vi "1-1 Constellations.vi"() -> ()   [LabVIEW 2019, in "AoC2022.lvlib"]
uses:
  AoC2022.lvlib
panel:
  out "Array":i32[][](array[numeric])
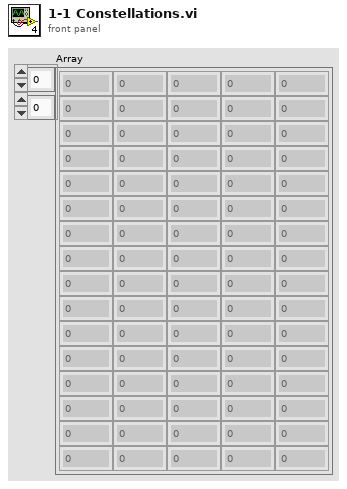
[diagram p1: front panel]
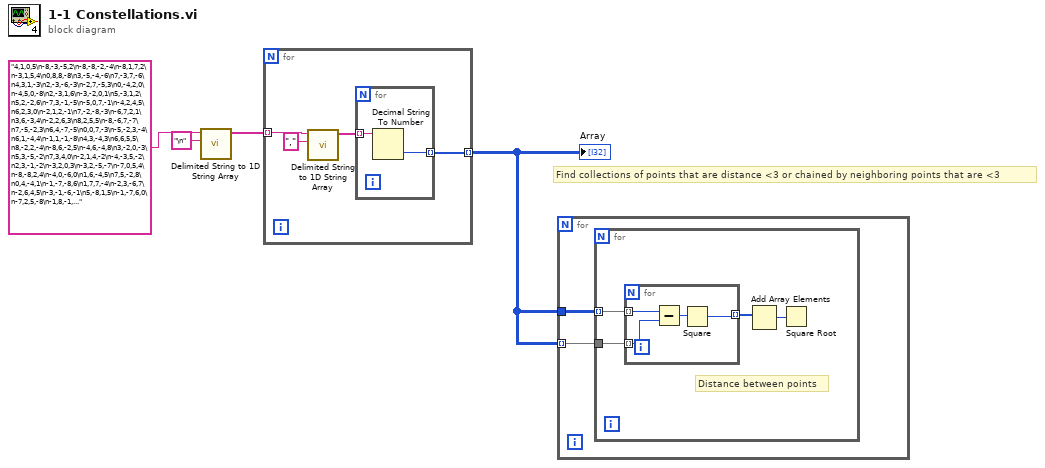
[diagram p0: block diagram]
diagram:
  # "Find collections of points that are distance <3 or chained by neighboring points that are <3"
  n1 = call <vilib>:"Delimited String to 1D String Array.vi"("delimiter"="\n", "delimited string"="4,1,0,5\n-8,-3,-5,2\n-8,-8,-2,-4\n-8,1,7,2\n-3,1,5,4\n0,8,8,-8\n3,-5,-4,-6\n7,-3,7,-6\n4,3,1,-3\n2,-3,-6,-3\n-2,7,-5,3\n0,-4,2,0\n-4,5,0,-8\n2,-3,1,6\n-3,-2,0,1\n5,-3,1,2\n5,2,-2,6\n-7,3,-1,-5\n-5,0,7,-1\n-4,2,4,5\n6,2,3,0\n-2,1,2,-1\n7,-2,-8,-3\n-6,7,2,1\n3,6,-3,4\n-2,2,6,3\n8,2,5,5\n-8,-6,7,-7\n7,-5,-2,3\n6,4,-7,-5\n0,0,7,-3\n-5,-2,3,-4\n6,1,-4,4\n-1,1,-1,-8\n4,3,-4,3\n6,6,5,5\n8,-2,2,-4\n-8,6,-2,5\n-4,6,-4,8\n3,-2,0,-3\n5,3,-5,-2\n7,3,4,0\n-2,1,4,-2\n-4,-3,5,-2\n2,3,-1,-2\n-3,2,0,3\n-3,2,-5,-7\n-7,0,5,4\n-8,-8,2,4\n-4,0,-6,0\n1,6,-4,5\n7,5,-2,8\n0,4,-4,1\n-1,-7,-8,6\n1,7,7,-4\n-2,3,-6,7\n-2,6,4,5\n-3,-1,-6,-1\n5,-8,1,5\n-1,-7,6,0\n-7,2,5,-8\n-1,8,-1,-1\n5,0,-2,0\n-1,-2,8,6\n-4,3,2,4\n-8,0,3,2\n7,7,-4,6\n4,7,-3,1\n5,-7,-3,0\n5,2,-3,8\n1,-3,-7,-3\n7,-5,2,7\n3,5,0,5\n3,1,-7,5\n-3,-2,7,-6\n1,0,8,-3\n-2,3,-1,6\n6,6,2,-5\n-8,-5,-5,7\n8,5,-6,6\n-2,6,-3,0\n6,1,-6,-6\n-5,7,-8,1\n-6,-5,0,2\n-3,0,1,-1\n1,5,7,4\n7,1,1,1\n7,-7,7,0\n5,8,0,7\n3,4,-2,-7\n-3,-8,8,0\n0,6,3,2\n7,-1,-5,-1\n2,-3,-1,3\n6,2,3,-7\n-3,-5,4,-3\n-6,-5,-7,4\n3,-3,-4,4\n3,7,-1,4\n6,0,-4,3\n3,-5,-2,-4\n-2,3,6,0\n2,5,5,8\n4,0,3,-5\n-2,1,3,-4\n-6,2,8,6\n4,-7,6,-6\n1,0,-7,8\n-2,-7,-6,3\n4,-1,6,4\n2,-2,0,-8\n8,7,0,7\n-5,6,-8,7\n-2,2,2,3\n3,4,6,5\n-6,0,0,-4\n-3,8,0,8\n-7,0,-3,-5\n-8,8,7,1\n7,0,6,4\n3,4,0,-8\n0,0,7,-8\n-6,1,-1,-5\n-1,0,4,-8\n-8,-1,-8,6\n7,3,6,0\n7,2,4,0\n5,-7,0,3\n0,3,0,-8\n-6,-7,-8,1\n6,0,-5,-4\n8,1,3,6\n-2,5,-7,2\n2,3,0,0\n-8,-2,0,-7\n0,0,1,-1\n0,-8,-3,4\n0,-7,-4,-7\n-6,2,-4,4\n-3,-6,-8,-8\n7,-3,-4,5\n-6,0,-5,-2\n2,-8,-3,-6\n2,0,1,-4\n2,-8,1,0\n-1,-5,-8,-4\n5,2,5,-3\n-8,-1,-2,-5\n7,0,1,-6\n0,-1,5,-5\n-6,4,8,-1\n-7,5,3,1\n-2,-5,5,8\n6,-2,8,7\n-4,-5,8,-4\n8,-8,1,6\n-6,4,2,-6\n0,-6,3,8\n-7,0,3,-5\n-3,-7,4,0\n8,-4,-8,6\n-1,-5,6,-4\n7,-5,-8,6\n2,-6,1,2\n-7,-8,7,3\n-7,1,-5,0\n6,4,4,-5\n5,1,-1,-4\n2,4,5,-1\n-2,-6,-7,0\n3,5,1,-5\n8,-8,-5,6\n-5,-4,6,5\n0,0,6,-2\n4,0,-6,-1\n3,8,-5,-2\n-2,8,1,8\n6,3,2,-4\n-3,-4,6,-8\n4,0,-6,2\n8,7,2,1\n-1,3,6,-5\n-1,7,-5,-2\n0,6,-2,1\n2,4,6,7\n-5,-4,4,-1\n5,7,-2,3\n4,8,0,-4\n6,-6,7,-7\n-5,-7,3,-2\n7,-3,7,0\n-4,2,-4,-5\n3,0,0,8\n8,-8,-1,5\n0,0,2,8\n4,0,-3,-3\n-4,6,8,0\n-6,6,-2,3\n0,0,-3,5\n-6,-8,4,-3\n-3,5,-5,7\n2,2,6,4\n-5,3,6,7\n-1,-7,7,2\n-7,-1,-8,6\n7,5,2,-2\n4,5,5,6\n0,3,5,6\n-3,-8,3,-1\n-2,3,-5,0\n1,1,-3,0\n6,-5,1,1\n0,-2,-3,3\n-6,-7,-1,-5\n3,-8,-3,-1\n-5,-4,4,-7\n0,6,-4,-1\n3,-5,0,-6\n5,0,-6,-4\n0,-5,-4,-8\n-2,5,1,-6\n-5,-2,-8,-2\n0,-2,-6,-6\n-5,-5,5,0\n7,6,-4,1\n8,4,0,7\n-1,6,6,-5\n0,8,-7,6\n-1,1,3,0\n0,0,-1,3\n8,0,-3,0\n0,-5,-2,1\n-3,7,-1,2\n2,3,-8,-7\n-8,-1,-4,-3\n8,7,-2,3\n6,-5,0,-6\n-7,8,1,0\n-5,-7,-6,-1\n0,-4,0,-8\n-3,8,0,2\n0,-1,4,-3\n-6,-1,2,1\n0,-4,-4,-2\n0,-1,-3,2\n-2,-3,-2,2\n-5,3,-8,5\n-4,2,5,-4\n1,5,4,3\n-8,4,-1,-4\n-6,-4,-7,0\n-7,5,-7,1\n1,2,5,0\n7,0,1,-8\n-7,7,4,-8\n8,4,7,-4\n4,5,0,4\n0,-6,7,4\n7,-8,2,7\n7,-1,-1,-8\n7,3,4,-6\n-4,0,1,-2\n5,5,0,-1\n8,6,8,-8\n-2,-4,4,2\n-7,4,2,4\n-1,3,-6,-5\n0,4,0,0\n-5,4,8,0\n6,6,8,-8\n5,-8,6,0\n-8,6,3,-7\n-1,7,0,5\n-2,-3,7,-3\n0,-3,7,2\n2,-3,-4,-6\n7,3,-7,-5\n7,5,7,-1\n-4,7,-1,8\n3,-3,5,0\n-4,-4,2,-2\n1,1,-4,0\n3,-1,6,0\n5,-5,5,-6\n5,-8,-1,5\n-2,-5,3,-7\n1,-1,0,-4\n7,2,-8,6\n7,2,-6,-5\n7,-2,-4,-6\n8,-3,3,1\n5,4,1,-6\n0,-8,-2,0\n0,-6,4,2\n8,1,4,3\n-4,7,0,0\n-3,1,-3,-4\n2,-1,-6,0\n-1,8,-4,-6\n-3,8,0,1\n7,0,4,-2\n-2,2,-8,-4\n8,2,3,2\n-1,-7,-6,7\n4,-5,0,5\n-3,4,8,-3\n6,0,-3,-3\n-5,5,-6,5\n3,8,-4,5\n7,0,7,-7\n-3,-3,-2,7\n0,-2,2,-6\n4,-1,7,-5\n8,-8,0,-6\n5,-6,-4,0\n-4,8,5,-2\n2,-8,-3,3\n2,0,1,-8\n-1,-3,-8,-1\n-3,-5,-2,0\n2,-5,1,-5\n8,3,0,-4\n-2,-8,0,-3\n-8,3,-7,-4\n6,-6,-1,2\n-1,5,-2,1\n-1,2,-3,-2\n-5,-6,7,-4\n4,-8,3,5\n0,-1,0,-1\n-6,5,8,1\n2,7,-3,0\n-6,6,-5,-5\n6,8,-2,6\n4,2,2,4\n-3,0,-8,0\n0,-3,-4,-5\n4,-1,0,0\n1,5,6,2\n-4,-7,7,0\n5,1,5,-5\n4,0,0,-2\n0,1,-2,-1\n5,-7,-5,7\n3,2,3,4\n0,0,-3,8\n5,2,-7,6\n2,5,-3,6\n-7,1,2,4\n1,4,-3,0\n-7,0,3,-4\n-5,1,-1,-4\n2,-8,-7,3\n2,3,-6,2\n-5,5,-6,-3\n0,5,8,2\n5,-4,-1,2\n-3,2,5,-6\n4,5,0,-3\n-6,-5,6,0\n0,-7,-2,-3\n-6,5,-6,0\n-7,3,3,-1\n6,3,-1,-2\n2,0,0,4\n0,-1,8,6\n-4,1,-4,-1\n7,-3,7,-1\n0,6,3,0\n-8,-4,-1,-4\n-1,-5,0,-8\n0,-5,-3,0\n0,-2,-2,6\n5,-7,5,-7\n5,-4,-6,-5\n0,-5,0,3\n7,-2,-1,8\n0,-1,-8,7\n-2,5,2,6\n-4,-4,-3,0\n-2,2,5,1\n2,-1,-7,7\n-2,-4,-6,-3\n4,0,-1,-4\n-8,8,-5,5\n5,-2,3,6\n6,-1,7,-7\n5,-5,6,-4\n7,7,-6,-6\n-5,8,-2,4\n1,6,-2,7\n0,2,3,2\n-5,-8,-5,-2\n5,-3,-7,-5\n4,5,6,4\n-4,-2,-1,-4\n4,-6,-2,-7\n-2,2,-1,-8\n-5,2,-4,5\n7,-6,-1,7\n0,3,-2,3\n-7,-3,8,8\n-7,6,-3,1\n-8,0,-2,1\n0,5,-6,0\n1,-6,-2,7\n0,-3,4,0\n8,4,5,-8\n2,-7,-6,4\n6,4,7,-5\n-5,6,-4,2\n0,-5,5,2\n-7,-8,2,4\n7,7,-5,6\n-7,5,2,5\n-6,-4,4,0\n0,-4,6,-2\n-4,4,7,6\n1,-3,-4,-6\n0,8,-8,-5\n0,2,1,0\n-5,-6,0,4\n-7,7,7,-7\n-8,3,6,-1\n7,3,-7,-2\n0,-8,2,-6\n8,3,-5,-1\n8,7,-6,-7\n-5,-3,6,7\n-6,-6,-7,-6\n3,-2,-8,-8\n-6,3,8,5\n4,3,8,6\n-7,6,-3,7\n3,7,5,5\n0,3,-6,4\n-6,-3,-8,2\n2,-7,6,0\n-1,3,-1,0\n-3,-4,4,8\n-8,-1,-5,4\n-4,-4,0,8\n0,7,5,4\n2,0,-4,2\n6,0,-5,5\n-8,0,-5,4\n6,-2,7,1\n5,-5,-3,8\n1,-5,0,-4\n-5,5,0,5\n-5,-3,8,-8\n-5,-2,5,6\n0,-6,-4,-4\n0,-1,1,-5\n0,0,6,-4\n4,-3,5,-4\n8,3,0,-6\n0,6,8,7\n4,2,-5,-5\n0,-1,0,-8\n-1,6,-2,-5\n-1,-5,-5,-7\n-3,-6,2,0\n0,0,1,3\n-7,3,0,0\n3,6,3,-3\n6,-8,-1,0\n7,-6,1,-7\n-8,-6,-8,0\n6,-7,5,4\n-1,2,4,2\n0,7,6,8\n0,-7,4,-5\n2,5,-6,2\n-8,-2,4,4\n5,1,-7,-7\n6,2,5,-3\n4,-5,-2,-4\n-2,2,-5,3\n8,0,4,8\n2,2,-6,4\n4,0,7,3\n-5,-6,6,4\n-6,0,-3,-1\n-1,8,-1,-8\n-7,-5,-3,-2\n3,3,-7,-3\n-6,4,-5,4\n8,-1,-3,7\n5,5,5,2\n0,0,1,0\n3,8,1,1\n6,6,-8,3\n-4,5,3,-6\n-3,8,4,6\n2,0,5,-4\n3,6,-5,5\n4,1,-8,0\n1,1,-3,-4\n8,-1,-8,3\n4,-6,-6,-7\n-1,0,-6,1\n0,2,8,-3\n-2,1,0,5\n-8,2,6,3\n-3,0,-8,7\n-6,-5,0,-6\n1,-7,1,-8\n-7,-8,3,0\n-6,4,-6,-7\n1,-2,4,0\n0,-3,-7,8\n-1,0,-2,0\n0,4,0,5\n-2,-1,-8,2\n1,-6,-2,-7\n6,-5,2,8\n-5,5,-2,-6\n3,-2,-3,-5\n8,2,-6,8\n0,-5,3,7\n8,7,-8,0\n-3,6,-6,8\n-6,5,7,3\n-2,-7,-7,-6\n-2,6,5,5\n0,2,-5,8\n3,-1,2,-4\n-8,-3,5,7\n0,3,-8,0\n8,-6,2,4\n8,-3,-4,-8\n7,-6,6,-3\n3,-7,-6,-2\n-6,3,3,-1\n4,0,0,5\n-3,-7,0,-7\n3,-4,-1,4\n5,-3,0,1\n5,-7,2,2\n-4,3,1,-1\n-3,4,-3,6\n7,1,0,-8\n-7,-3,-2,-8\n4,0,4,1\n-2,0,-4,-3\n1,-4,0,-6\n-7,-2,8,5\n0,2,-5,-5\n5,0,0,2\n-3,0,-6,-4\n-5,0,0,1\n-3,3,0,-1\n-1,-6,0,-5\n6,-1,-5,-6\n-8,-5,-8,0\n0,4,5,-6\n5,4,-8,6\n6,-7,-2,-4\n0,6,5,-4\n-6,-2,-2,0\n-2,2,-1,-5\n1,4,0,-5\n5,-3,2,4\n-8,8,-3,3\n-3,1,-4,-3\n7,-2,2,-5\n-6,-3,-5,5\n7,7,0,2\n-4,0,-2,-1\n1,-4,3,5\n-2,-2,7,5\n-4,-7,-5,-4\n-1,0,4,3\n1,-4,-4,3\n-6,-7,8,1\n-2,4,5,-2\n-5,-8,-5,5\n8,-3,5,6\n0,8,-4,3\n-7,0,-5,0\n-6,1,-6,-4\n-4,-1,0,-8\n3,7,-6,0\n3,6,6,-6\n0,3,0,1\n1,1,8,0\n8,-8,-5,-8\n5,-2,5,-3\n-4,-4,-3,-2\n0,3,-7,-6\n7,-8,0,1\n-5,4,7,4\n-4,3,-5,7\n-4,-2,-8,-3\n-1,-6,0,-7\n-1,-7,7,-6\n-1,-3,0,-2\n-3,-5,7,5\n-1,0,-5,0\n-7,5,-3,-5\n0,-5,8,1\n8,6,-8,8\n1,-7,4,6\n0,0,0,-8\n-4,7,-6,-2\n-7,-7,-6,-4\n1,-7,8,-3\n4,4,-3,0\n-8,6,0,5\n-3,1,6,-3\n-8,-8,8,-3\n4,-4,-7,-8\n6,7,2,5\n0,8,-3,0\n8,4,-4,-7\n0,0,3,0\n1,-3,-3,-4\n-4,-6,-3,3\n0,6,-2,-3\n6,-6,-5,-5\n7,6,8,-4\n7,-1,6,-6\n3,0,1,-6\n7,6,-8,0\n0,-2,4,0\n2,1,0,-8\n3,-5,5,-6\n-4,-8,7,-8\n1,-4,-3,-7\n-4,-3,-5,-4\n0,8,-8,4\n3,-3,3,-7\n0,-7,1,4\n6,1,1,4\n2,1,-5,4\n-6,-8,0,3\n7,2,-6,0\n-4,6,0,-6\n4,7,-8,0\n1,-1,5,-1\n-4,0,-7,-1\n-7,8,4,0\n-2,0,4,3\n-6,0,-2,-4\n6,-4,1,0\n-1,5,7,5\n8,-4,8,0\n1,-6,0,-4\n2,2,0,2\n6,8,7,-5\n-3,-5,-4,3\n5,1,-4,-8\n-4,-7,3,0\n5,-6,3,5\n-5,2,1,-5\n3,3,-2,8\n-1,0,7,-4\n-3,-3,-5,0\n-7,0,-3,-3\n-6,-5,4,8\n1,0,-5,2\n-3,-8,-2,-6\n-8,8,0,-7\n4,-6,-8,-8\n-7,1,1,1\n2,0,-6,-3\n5,6,-5,5\n0,4,-3,6\n0,-1,-3,-5\n2,-3,-5,-4\n5,-1,0,-5\n6,-7,-4,1\n-6,-8,8,-2\n-8,7,-2,-2\n8,4,-8,7\n8,-3,-6,6\n-4,-3,4,5\n-2,8,4,-4\n7,-7,3,0\n4,-3,6,0\n-6,-7,4,5\n-6,4,-5,0\n1,1,-1,0\n-2,0,8,6\n3,-3,5,-8\n-6,1,-5,0\n-4,0,1,5\n8,-2,-3,2\n-4,-5,7,3\n-7,-4,5,5\n-3,7,0,4\n-5,0,3,3\n-5,8,-5,4\n6,0,-6,1\n0,3,3,8\n0,-3,-8,-8\n-4,-4,3,0\n-1,0,8,-8\n0,-3,-1,3\n-3,3,-3,6\n-1,-8,-3,-1\n4,2,-2,0\n7,5,-4,-7\n-4,-6,-1,7\n7,4,8,6\n-6,-6,3,-6\n-6,0,8,1\n-7,-2,0,4\n8,-8,-4,-3\n0,7,2,-6\n8,5,-8,-4\n5,3,3,3\n3,-6,-7,2\n6,2,0,3\n-5,5,-4,0\n0,-5,0,-4\n0,-5,6,-1\n2,2,4,-5\n7,-3,0,7\n0,5,-4,-5\n-3,5,-7,-3\n0,-2,5,2\n-3,8,-1,-6\n8,-8,8,-5\n4,-2,0,-2\n1,1,2,0\n-7,-2,-6,-4\n-5,1,7,6\n0,0,-7,2\n-7,-2,-1,-3\n6,2,-4,1\n-3,0,2,-3\n0,-3,2,-1\n3,7,-4,0\n-1,0,1,-1\n-6,8,-6,0\n-4,-3,-1,4\n5,-7,3,8\n6,8,-3,5\n1,2,-3,5\n0,5,1,4\n-4,2,3,-3\n3,-3,-7,-4\n8,0,0,-7\n8,2,7,3\n-6,-8,7,3\n-1,0,4,-2\n4,4,-6,6\n5,0,-3,4\n-5,-4,8,-8\n0,-1,-1,0\n6,-2,-1,4\n-4,0,-6,-8\n2,6,0,6\n0,0,-2,-6\n8,-1,-6,0\n8,1,-6,-1\n-4,1,6,-3\n-5,-1,-6,-8\n8,0,-1,2\n3,0,7,6\n-1,-2,5,-2\n3,-2,7,1\n-4,1,7,-3\n-5,-5,6,7\n-5,-1,7,-4\n7,1,-3,-5\n-8,1,2,-5\n-4,0,-6,4\n-3,-1,-3,4\n-8,5,0,7\n0,-2,8,-5\n-3,8,4,1\n8,2,2,4\n-1,-3,5,-8\n7,3,2,8\n0,8,0,3\n3,-4,-8,4\n1,1,-3,-1\n0,3,2,0\n7,8,-1,1\n-2,4,-6,0\n2,4,-8,-8\n-5,4,-3,7\n-2,5,4,-7\n-3,-3,0,-1\n1,-3,-7,6\n0,7,-4,-4\n0,-4,-8,0\n8,0,2,3\n-2,-4,5,-1\n-3,6,5,1\n-7,-4,-5,5\n1,2,-2,7\n-6,3,5,-6\n-6,-2,6,2\n3,-7,-2,0\n7,-7,-6,1\n-3,0,1,-6\n-1,-3,-7,-8\n6,6,-6,-8\n2,8,-5,-3\n2,6,6,-4\n7,0,0,-4\n-7,-4,3,8\n-8,4,-6,5\n8,-7,0,-4\n-7,8,0,-1\n-4,8,-5,-5\n-8,-8,-5,-4\n0,4,5,-5\n4,0,-7,-5\n-2,-2,7,-4\n-2,-8,0,-8\n4,8,8,-6\n4,1,-4,1\n-8,-8,2,-1\n5,5,4,1\n-2,2,-8,-8\n-4,0,6,-2\n6,4,-6,4\n7,-3,3,0\n0,4,6,-4\n1,-1,0,0\n2,-5,2,4\n-3,3,-4,-4\n-3,-4,-8,-5\n0,0,-1,5\n-2,-8,7,-3\n4,-2,7,-2\n-3,6,-8,0\n8,4,8,4\n7,-8,1,-5\n-3,8,2,8\n2,6,0,-7\n6,-8,0,0\n2,-4,-8,6\n-3,-1,-8,5\n-8,-7,-7,8\n6,4,3,-2\n7,-5,6,-8\n-5,2,4,8\n5,-2,1,-5\n6,2,-8,-8\n-3,-6,1,0\n-5,-8,8,2\n3,4,-4,4\n-1,-5,7,-3\n-6,-8,-6,3\n-6,-5,-2,7\n2,-5,8,-1\n1,6,-2,-1\n3,-4,1,4\n-3,-8,-5,0\n6,4,8,5\n-4,0,5,-2\n2,-8,-7,-2\n-2,8,-2,1\n5,6,1,6\n-5,4,-4,-8\n-8,1,-1,7\n7,-4,0,-1\n2,8,8,1\n7,4,-4,-8\n0,-2,-5,6\n-3,-1,-4,4\n8,7,-7,1\n-5,-8,-4,-8\n-8,-3,8,-5\n4,1,5,6\n8,0,6,-3\n8,-7,7,0\n-2,7,1,-3\n-3,-7,5,-5\n0,-7,-2,1\n0,3,-3,2\n-1,1,4,6\n-1,-4,3,-7\n-2,2,4,6\n-2,-7,-1,7\n3,-7,2,-4\n0,5,8,1\n-2,-8,-7,-6\n-1,8,-6,3\n-1,4,0,-1\n6,4,3,5\n-3,-3,-8,-1\n2,-1,5,-3\n3,3,7,-6\n3,-4,-1,0\n0,-1,-2,-4\n-5,4,4,2\n-8,5,-6,-3\n0,4,5,0\n3,-5,-2,1\n-8,-3,5,5\n3,0,4,-2\n-3,-8,4,-2\n0,6,-7,-2\n8,-2,6,-6\n5,7,5,7\n-3,-3,-6,5\n-8,-7,-2,0\n4,-1,-4,3\n-5,5,-8,-6\n2,4,5,6\n-2,1,-6,-1\n2,-2,5,7\n0,-3,-3,4\n-5,7,1,-5\n-5,-2,0,0\n-4,-3,0,2\n-4,-6,0,-7\n0,-1,6,2\n-3,4,6,-6\n3,-2,6,2\n6,-4,-8,4\n4,-2,-6,0\n1,7,-1,3\n0,4,8,5\n-1,4,2,-5\n0,-2,5,-6\n5,6,2,-5\n-1,-8,2,-8\n-4,1,6,-7\n-2,1,-5,0\n-8,7,0,5\n-4,-7,-3,3\n1,-6,5,7\n-1,3,8,3\n-3,3,-4,-1\n2,-7,0,0\n-7,3,1,-1\n8,5,-8,0\n-4,-5,6,0\n-6,0,8,-5\n6,5,8,-6\n3,-7,1,-5\n-7,-4,6,-2\n-6,0,6,-7\n-4,-6,-6,-8\n0,-6,-7,-1\n7,-5,-1,3\n7,-7,-1,-3\n1,5,6,-5\n-1,-2,1,3\n0,5,1,7\n8,-5,-1,7\n7,2,0,-1\n-1,0,7,8\n-6,0,7,6\n3,-3,-8,4\n0,8,-1,8\n-7,2,-5,5\n3,-4,-2,7\n1,0,4,-3\n3,-2,2,0\n0,2,6,-7\n-3,-5,1,-6\n8,-1,0,-5\n0,-5,-5,8\n-1,2,4,-8\n0,-7,-8,-1\n0,-7,-2,-6\n-4,-4,-2,-3\n0,0,4,3\n-3,-3,3,0\n-2,-6,5,-5\n-3,7,2,-4\n4,-6,-7,4\n5,0,0,-5\n4,4,-7,0\n6,-6,-8,3\n3,-8,-8,5\n-2,2,-7,-2\n8,8,0,8\n0,6,-4,5\n7,0,-8,-5\n-5,3,1,1\n-2,4,4,0\n0,7,8,6\n7,-1,-7,2\n-4,0,-1,8\n0,-3,-2,0\n0,-6,-7,0\n7,6,-2,-7\n-3,-5,3,-6\n-4,-6,4,1\n3,6,-4,1\n-4,-8,-7,7\n6,0,-5,0\n6,8,0,7\n4,0,5,-3\n-4,-5,1,0\n3,5,6,3\n-7,-5,-7,8\n1,5,6,7\n5,-2,1,8\n-3,3,8,-4\n3,-4,-6,-7\n-3,1,-8,-3\n1,-2,7,4\n-6,-3,-2,3\n2,-5,-5,-6\n0,-8,5,-3\n6,4,-8,0\n0,3,6,-1\n-3,7,-7,-6\n-8,-6,-3,-3\n0,-7,8,-2\n2,-1,-3,8\n0,-7,0,1\n-7,5,4,6\n3,6,-4,2\n7,2,2,0\n0,-3,0,4\n1,-2,0,-1\n0,2,-3,-1\n1,-2,-4,4\n3,6,-2,1\n-8,-2,1,3\n-1,8,-6,5\n-4,-8,4,2\n-7,-2,0,7\n3,3,4,7\n0,-1,0,8\n-7,-5,8,5\n3,-1,8,8\n-6,7,-1,7\n0,8,2,-7\n-5,2,-5,0\n4,-4,-5,0\n-2,3,3,7\n4,7,-4,0\n7,-6,-5,-4\n7,-2,6,-5\n0,-8,2,3\n0,0,0,-5\n0,-1,-2,7\n3,0,1,6\n-8,-4,-2,-4\n0,0,0,3\n8,-6,5,0\n-6,8,2,2\n-5,-2,0,-1\n7,-4,1,-5\n8,-3,-4,-5\n2,-5,-5,0\n-8,-7,0,-6\n2,-2,-4,0\n0,-5,4,-5\n0,2,-4,4\n-3,-3,-2,0\n-4,5,4,-3\n0,0,0,2\n-4,-3,3,-5\n7,-6,-6,7\n-4,-3,-5,-8\n-3,-6,-7,-4\n-4,-5,7,-4\n-8,0,7,-4\n-1,5,-1,6\n5,7,5,6\n-5,3,2,7\n-6,7,-4,-5\n8,-8,-4,4\n8,3,-1,-3\n-1,0,4,-5\n0,-4,5,5\n-2,7,5,0\n-4,7,7,5\n4,6,3,0\n-4,-7,7,-3\n-4,7,1,-6\n0,1,-4,-8\n-7,-4,5,-7\n-4,0,-3,5\n1,8,4,-8\n0,0,6,7\n-1,-3,-3,-7\n-8,-3,-8,0\n4,-2,8,6\n0,2,-5,5\n1,5,-6,4\n-8,7,0,7\n8,-1,-8,-6\n0,3,-3,-8\n-5,6,3,-7\n6,4,5,6\n-5,3,4,-2\n-5,0,-2,0\n4,7,8,6\n2,-8,-5,8\n1,3,3,-3\n3,-7,-6,7\n1,3,5,3\n-1,4,7,-6\n3,-4,5,1\n3,6,4,7\n4,0,-7,3\n-1,-8,7,-6\n2,-1,-2,8\n2,2,-5,8\n-2,1,-1,3\n0,-8,0,2\n7,8,-4,6\n3,3,2,-5\n-7,-3,-4,6\n3,3,-8,3\n5,0,-7,3\n-8,-4,0,6\n0,1,5,-5\n4,-5,8,-7\n-6,-7,3,1\n8,-6,-2,0\n8,-3,-5,4\n0,2,-5,0\n4,2,-1,0\n2,8,-4,5\n0,-1,7,-2\n7,-5,-4,0\n-1,-5,5,5\n5,-6,2,-4\n-2,-7,5,2\n-1,-3,5,2\n-1,0,4,-1\n-8,2,-6,3\n-3,0,4,1\n0,0,4,-3\n2,-7,-5,0\n-5,1,7,8\n2,0,-4,-8\n2,7,1,6\n3,0,3,5\n0,-7,-3,6\n1,4,-1,7\n4,-3,6,-3\n-6,5,0,7\n-6,3,-8,1\n-4,-4,-1,4\n-4,-4,2,3\n6,-1,-8,1\n3,5,-6,1\n0,2,-2,6\n1,-8,3,-6\n-6,5,8,-1\n-6,7,2,0\n-4,-2,6,6\n4,2,-5,3\n1,6,6,7\n5,-1,-8,7\n6,-1,1,-5\n7,3,-3,-4\n-7,-2,0,8\n3,2,0,8\n8,4,0,6\n7,0,4,-4\n-3,-8,8,2\n1,-2,2,-8\n-6,-6,-5,-5\n-8,6,6,-7\n3,-6,2,-6\n-8,6,5,1\n3,-3,3,-3\n2,-7,5,-5\n0,2,2,7\n4,-2,5,5\n8,4,7,-2\n-7,-7,-8,-7\n5,0,-7,-8\n1,8,6,-8\n-5,5,2,6\n4,5,7,-2\n-2,-2,8,7\n0,-3,-8,8\n3,7,2,-4\n-5,1,0,6\n0,6,-2,-7\n-8,4,-5,2\n-7,6,-8,3\n6,6,-8,-4\n3,7,-8,-3\n-7,-6,-1,-5\n-5,6,-6,0\n-2,5,6,4\n-8,-5,1,-4\n8,1,4,-2\n0,2,-4,1\n-6,0,2,-5\n-4,-4,1,6\n-1,-3,-5,7\n3,4,6,2\n-8,0,-2,-5\n8,0,8,0\n1,-1,-1,-3\n-7,0,2,4\n-8,1,4,0\n0,8,1,-3\n8,8,0,7\n8,-1,8,5\n0,1,8,-2\n6,8,0,1\n6,-1,-5,-8\n3,-4,-3,5\n-1,-2,3,4\n-4,-8,3,5\n5,4,-2,-4\n3,0,-5,2\n-7,3,4,8\n1,0,-8,7\n-2,0,4,-6\n-3,4,-3,0\n-6,-6,-3,3\n-2,2,0,6\n2,4,-2,-6\n-7,0,-8,-4\n-8,-3,7,-6\n7,6,4,-7\n-8,0,0,-7\n-1,1,-5,0\n5,6,-2,3\n-6,0,0,3\n-3,-6,5,-2\n-4,1,2,-6\n-3,-1,-3,8\n1,2,4,-1\n-7,8,0,5\n-8,2,-1,-5\n-4,-7,-8,-1\n-8,-4,0,-2\n4,-5,-3,6\n0,-7,2,-7\n0,6,-8,-7\n-4,7,-6,7\n-7,0,-3,-6\n6,-4,-2,1\n3,-4,4,-1\n8,4,-7,-2\n7,-8,2,8\n3,1,-8,1\n2,-4,-4,-6\n8,-4,2,-1\n3,-3,-2,2\n5,-3,8,6\n7,-2,-6,-3\n4,3,0,-8\n4,0,-4,8\n6,0,-4,-5\n-3,2,-8,4\n5,5,-5,-1\n-8,7,-1,1\n1,5,-7,-4\n-2,-7,6,4\n0,6,0,0\n-7,-5,-5,-6\n4,8,0,-1\n4,7,-6,6\n5,-3,2,0\n-2,-8,4,-5\n-3,-7,-4,8\n8,6,3,-5\n-7,-2,8,-6\n0,-6,-8,-5\n-5,0,2,4\n-3,0,6,6\n-3,-6,4,-5\n2,-6,0,8\n5,-6,2,-1\n-3,2,-1,3\n-1,7,0,-1\n6,4,-3,6\n0,0,-6,-1\n-5,-2,4,-3\n0,-1,2,-4\n4,4,5,-8\n-7,1,-2,0\n4,0,-1,6\n2,0,0,-3\n4,8,7,2") -> ("string array"=w2:string[])  [unwired: 9 in]
  n2 = for {
    tunnel: w2 -> [w8] mode=indexing
    tunnel: [w5] -> w1 mode=indexing
    n3 = call <vilib>:"Delimited String to 1D String Array.vi"("delimiter"=",", "delimited string"=w8) -> ("string array"=w6:string[])  [unwired: 9 in]
    n4 = for {
      tunnel: w6 -> [w10] mode=indexing
      tunnel: [w9] -> w5 mode=indexing
      n5 = Decimal String To Number(string=w10) -> (number=w9:i32)  [unwired: 2 in, 1 out]
    }
  }
  "Array" <- w1
  n6 = for {
    tunnel: w1 -> [w11] mode=indexing
    tunnel: w1 -> [w12]
    n7 = for {
      tunnel: w12 -> [w16] mode=indexing
      tunnel: w11 -> [w15]
      # "Distance between points"
      n8 = for {
        tunnel: w16 -> [w20] mode=indexing
        tunnel: w15 -> [w19] mode=indexing
        tunnel: [w17] -> w14 mode=indexing
        n9 = Subtract(x=w20, y=w19) -> (x-y=w18:i32)
        n10 = Square(x=w18) -> (x^2=w17:i32)
      }
      n11 = Add Array Elements(numeric array=w14) -> (sum=w13:i32)
      n12 = Square Root(x=w13) -> ()  [unwired: 1 out]
    }
  }
